vi "Save image.vi"(8 "Ring":u16(ring) items=["jpg", "png"], 11 "image data":T1) -> ()   [LabVIEW 2020]
doc: "With this SubVi image from chart can be saved do files - jpg or bmp"
uses:
  <vilib>/picture/picture.llb/imagedata.ctl
panel:
  in  "image data 2":T1
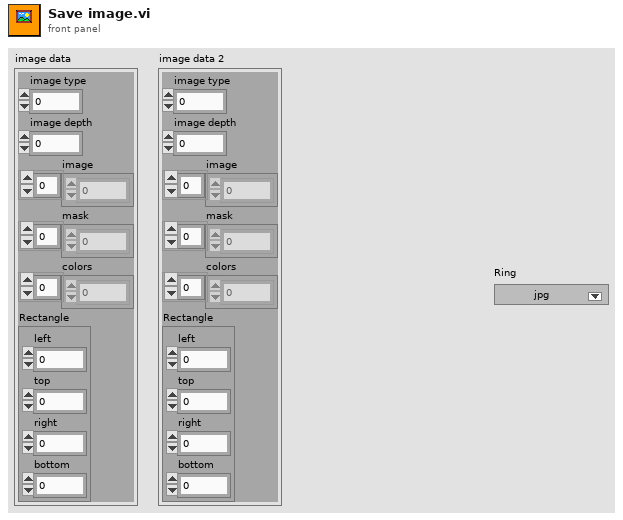
[diagram p1: front panel]
types:
  T1 = typedef "imagedata.ctl" = cluster{"image type":i32, "image depth":i32, "image":u8[], "mask":u8[], "colors":u32[], "Rectangle":cluster{"left":i16, "top":i16, "right":i16, "bottom":i16}}
  T2 = enum16{"open", "replace", "create", "open or create", "replace or create", "replace or create with confirmation"}
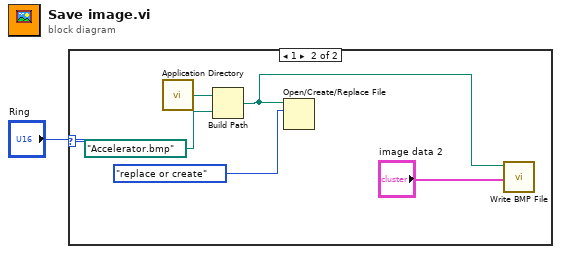
[diagram p0: block diagram]
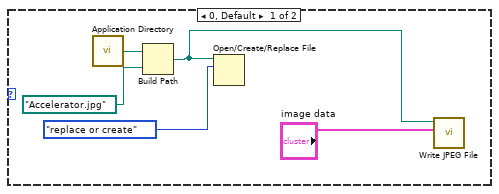
[diagram p2: hidden frame]
diagram:
  n1 = case shown="1" "Ring" {
    frame 0, Default {
      n2 = call <vilib>:"Application Directory.vi"() -> ("Application Directory"=w6:path)
      n3 = Build Path(base path=w6, name or relative path=path "Accelerator.jpg") -> (appended path=w5:path)
      n4 = Open/Create/Replace File(file path (use dialog)=w5, operation (0:open)=T2."replace or create") -> ()  [unwired: 4 in, 3 out]
      n5 = call <vilib>:"Write JPEG File.vi"("image data"="image data", "path to JPEG file"=w5) -> ()  [unwired: 8 in, 2 out]
    }
    frame 1 {
      n6 = call <vilib>:"Application Directory.vi"() -> ("Application Directory"=w11:path)
      n7 = Build Path(base path=w11, name or relative path=path "Accelerator.bmp") -> (appended path=w10:path)
      n8 = Open/Create/Replace File(file path (use dialog)=w10, operation (0:open)=T2."replace or create") -> ()  [unwired: 4 in, 3 out]
      n9 = call <vilib>:"Write BMP File.vi"("image data"="image data 2", "path to BMP file"=w10) -> ()  [unwired: 8 in, 2 out]
    }
  }
